vi "Simulation Statechart.vi"(5 "firstStep?":bool, 7 "enableVisualization?":bool=TRUE, 8 "error in":errorcluster, 10 "sensors":T1 {"Kobuki Sensors"."Charger Source" items=["DISCHARGING"=0, "DOCKING_CHARGED"=2, "DOCKING_CHARGING"=6, "ADAPTER_CHARGED"=18, "ADAPTER_CHARGING"=22]; "accelerometer"."z axis (g)" format="%.3f"; "accelerometer"."y axis (g)" format="%.3f"; "accelerometer"."x axis (g)" format="%.3f"}) -> (0 "error out":errorcluster, 1 "Diagram Display":picture, 2 "sensors":T1 {"Kobuki Sensors"."Charger Source" items=["DISCHARGING"=0, "DOCKING_CHARGED"=2, "DOCKING_CHARGING"=6, "ADAPTER_CHARGED"=18, "ADAPTER_CHARGING"=22]; "accelerometer"."z axis (g)" format="%.3f"; "accelerometer"."y axis (g)" format="%.3f"; "accelerometer"."x axis (g)" format="%.3f"})   [LabVIEW 2017]
uses:
  shared/Sensors.ctl
  shared/Accelerometer.ctl
  Kobuki/KobukiSensors.ctl
  Kobuki/Kobuki Bumps and WheelDrops.ctl
  Kobuki/Kobuki Buttons.ctl
  Statechart.lvsc/StatechartState.ctl
  Statechart.lvsc/State.ctl
  Statechart.lvsc/CompanionDiagram.vi/48/SC Main.vi
  Statechart.lvsc/CompanionDiagram.vi/48/Upd State.vi
  Statechart.lvsc/CompanionDiagram.vi/48/Trans Graph0.vi
  Statechart.lvsc/CompanionDiagram.vi/48/EnterGraphCore.vi
  Statechart.lvsc/CompanionDiagram.vi/48/Trans Graph1.vi
  Statechart.lvsc/CompanionDiagram.vi/48/Trans Graph2.vi
  Statechart.lvsc/CompanionDiagram.vi
  shared/Wrap Angle.vi
  Statechart.lvsc/Trigger.ctl
  <vilib>/Statechart/Infrastructure/RTStatechart/RunTime SCN.xnode
  Statechart.lvsc/Inputs.ctl
  Statechart.lvsc/Outputs.ctl
  Statechart.lvsc
panel:
  # "Electrical: charging, battery, OI mode"
  # "Sensors: bump, cliff, button, wheel drop"
  # "Motors:"
  # "Inertia"
  # "Electrical: charging, battery, OI mode"
  # "Sensors: bump, cliff, button, wheel drop"
  # "Motors:"
  # "Inertia"
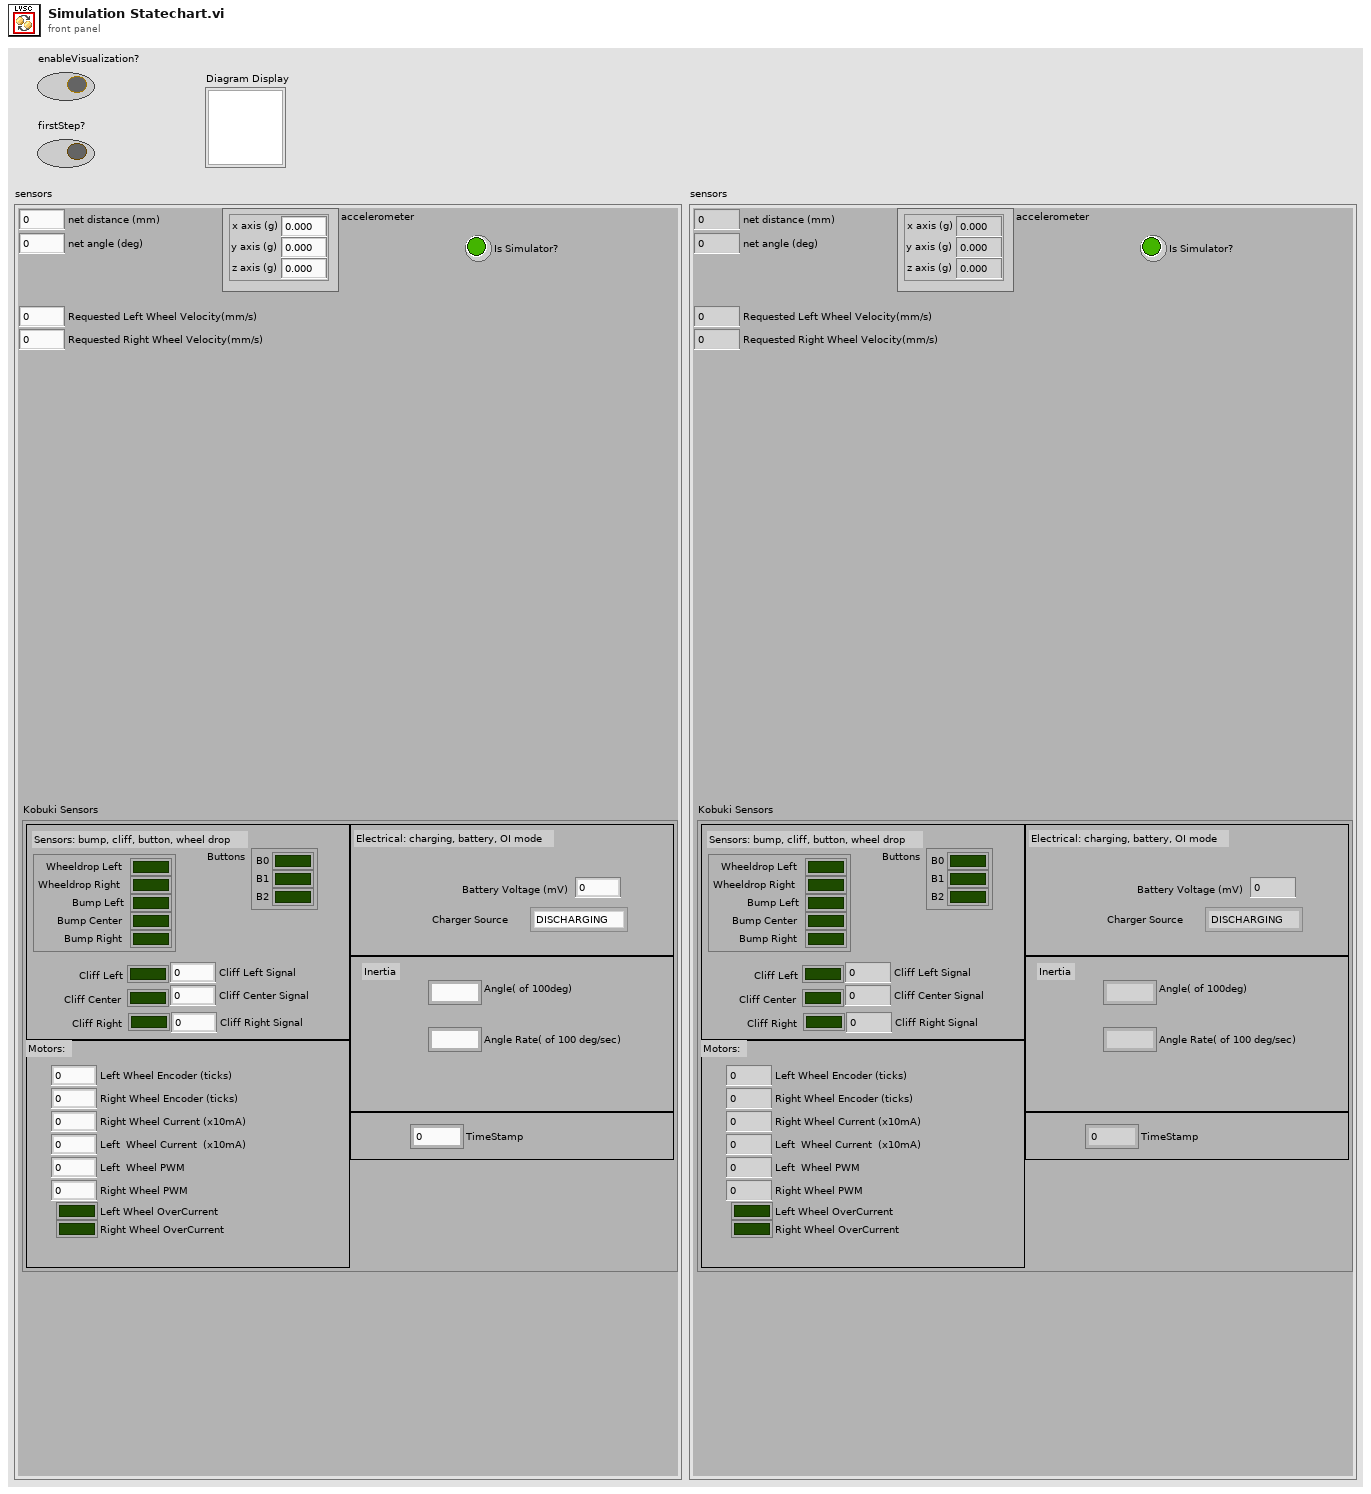
[diagram p1: front panel]
types:
  T1 = typedef "Sensors.ctl" = cluster{"net distance (mm)":i32, "net angle (deg)":i32, "accelerometer":T2, "Is Simulator?":bool, "Kobuki Sensors":T3, "Requested Left Wheel Velocity(mm/s)":i32, "Requested Right Wheel Velocity(mm/s)":i32}
  T2 = typedef "Accelerometer.ctl" = cluster{"x axis (g)":dbl, "y axis (g)":dbl, "z axis (g)":dbl}
  T3 = typedef "KobukiSensors.ctl" = cluster{"Bumps + Wheel Drops":T4, "Cliff Left":bool, "Cliff Center":bool, "Cliff Right":bool, "Cliff Left Signal":u16, "Cliff Center Signal":u16, "Cliff Right Signal":u16, "Buttons":T5, "Left Wheel Encoder (ticks)":u16, "Right Wheel Encoder (ticks) ":u16, "Left  Wheel PWM":i8, "Right Wheel PWM":i8, "Left Wheel OverCurrent":bool, "Right Wheel OverCurrent ":bool, "Right Wheel Current (x10mA)":i16, "Left  Wheel Current  (x10mA)":i16, "TimeStamp":u16, "Battery Voltage (mV)":i16, "Angle( of 100deg)":i16, "Angle Rate( of 100 deg/sec)":i16, "Charger Source ":i8}
  T4 = typedef "Kobuki Bumps and WheelDrops.ctl" = cluster{"Wheeldrop Left":bool, "Wheeldrop Right":bool, "Bump Left":bool, "Bump Center":bool, "Bump Right":bool}
  T5 = typedef "Kobuki Buttons.ctl" = cluster{"B0":bool, "B1":bool, "B2":bool}
  T6 = typedef "Statechart.lvsc/StatechartState.ctl" = T7[]
  T7 = typedef "Statechart.lvsc/State.ctl" = enum16{"NI.SC.Initial", "NI.SC.History", "NI.SC.ShallowHistory", "NI.SC.Terminal", "Pause", "Run", "Pause\\Detect Play Button\\Pause;\nWait for\nbutton\nrelease", "Pause\\Detect Play Button\\Unpause;\nwait for\nbutton release", "Pause\\Detect Play Button\\Unpause;\nwait for\nbutton press", "Run\\Run Mode\\Turn", "Run\\Run Mode\\Drive"}
  T8 = typedef "Statechart.lvsc/Outputs.ctl" = cluster{"Left Wheel Speed (mm/s)":i16, "Right Wheel Speed (mm/s)":i16}
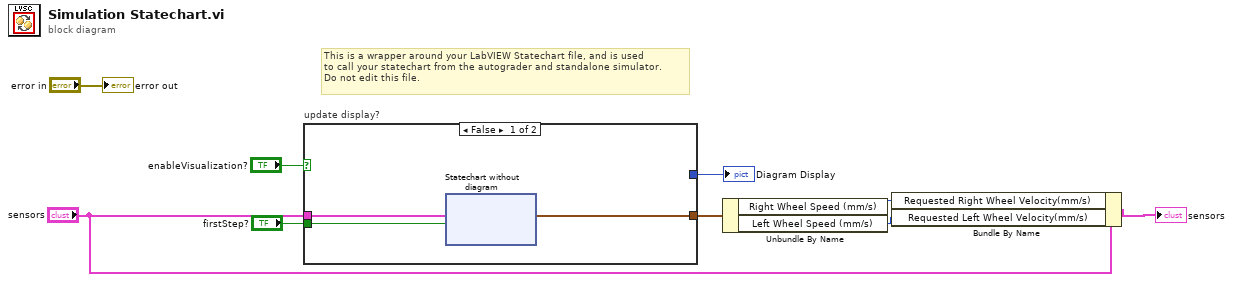
[diagram p0: block diagram]
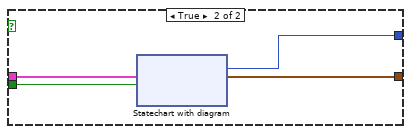
[diagram p2: hidden frame]
diagram:
  # "This is a wrapper around your LabVIEW Statechart file, and is used\nto call your statechart from the autograder and standalone simulator.\nDo not edit this file."
  n1 = case "update display?" shown="False" "enableVisualization?" {
    tunnel: "sensors" -> [w10 w18]
    tunnel: [w11 w21] -> w9
    tunnel: "firstStep?" -> [w12 w20]
    tunnel: [_ w19] -> w8
    frame False {
      n2 = xnode "Statechart without diagram"("Init?"=w12, "Inputs"=w10) -> ("Outputs"=w11:T8)  [unwired: 1 in, 1 out]
    }
    frame True {
      n3 = xnode "Statechart with diagram"("Init?"=w20, "Inputs"=w18) -> ("Outputs"=w21:T8, "Diagram Display"=w19:picture)  [unwired: 2 in, 1 out]
    }
  }
  "Diagram Display" <- w8
  n4 = Unbundle By Name(w9) -> ("Right Wheel Speed (mm/s)"=w1:i16, "Left Wheel Speed (mm/s)"=w2:i16)
  n5 = Bundle By Name(cluster="sensors", "Requested Right Wheel Velocity(mm/s)"=w1, "Requested Left Wheel Velocity(mm/s)"=w2) -> (→"sensors":T1)
  "error out" <- "error in"
